vi "MouseScrollAction.vi"(0 "XYGraph输入":refnum<vi>, 1 "Ynum":i32=8, 2 "Coords":T2, 3 "Delta":i32, 4 "PlatMods":T1, 5 "ZoomMode":u16) -> ()   [LabVIEW 2015]
uses:
  <vilib>/Utility/miscctls.llb/LVPoint32TypeDef.ctl
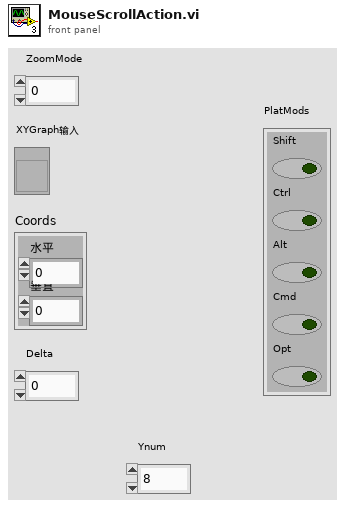
[diagram p1: front panel]
types:
  T1 = cluster{"Shift":bool, "Ctrl":bool, "Alt":bool, "Cmd":bool, "Opt":bool}
  T2 = typedef "LVPoint32TypeDef.ctl" = cluster{"Horizontal":i32, "Vertical":i32}
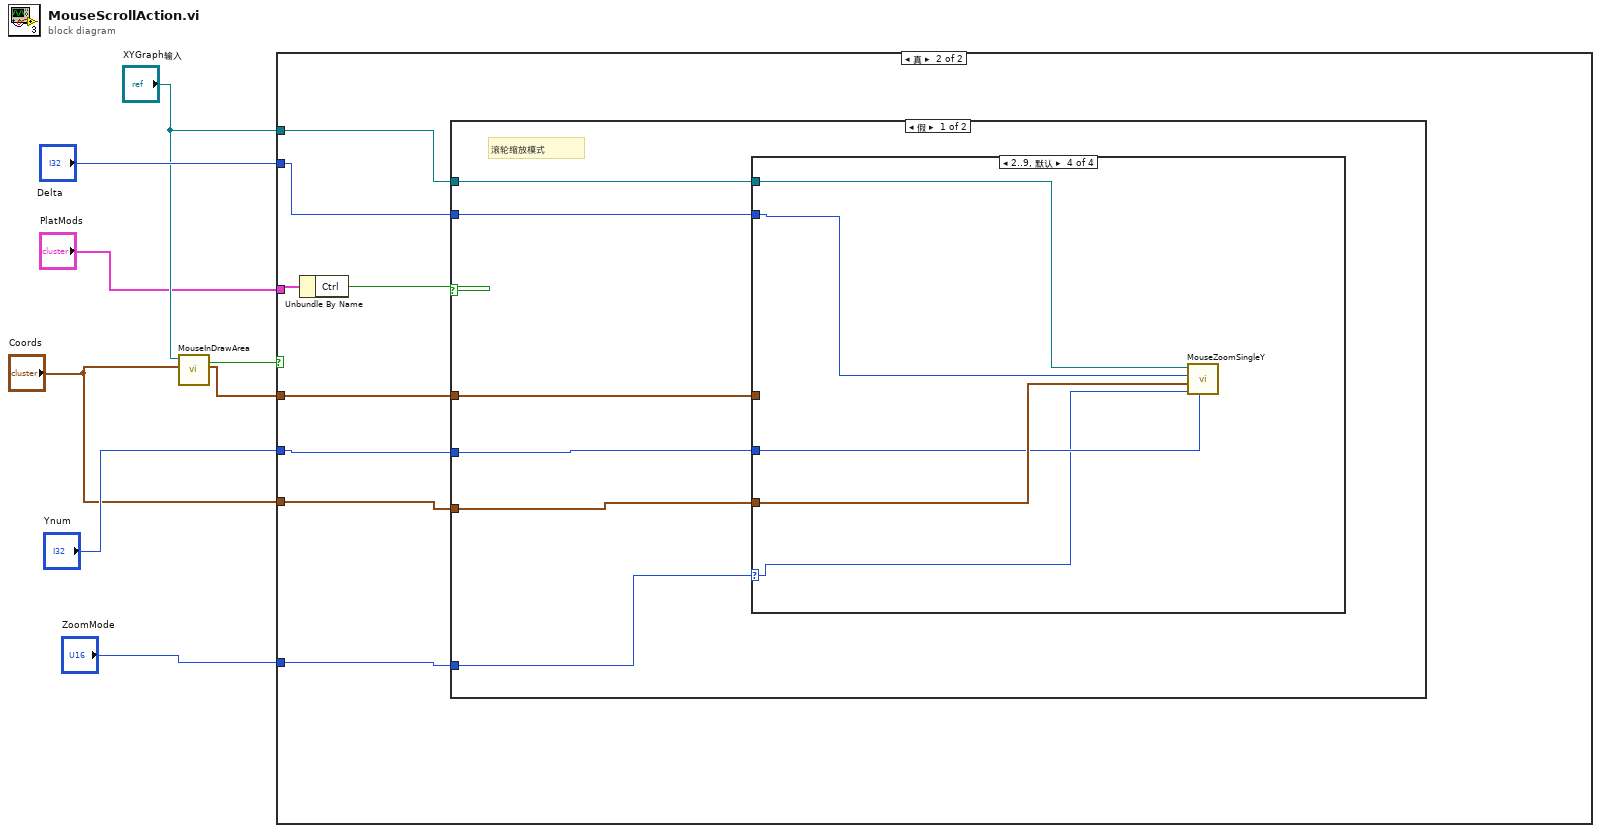
[diagram p0: block diagram]
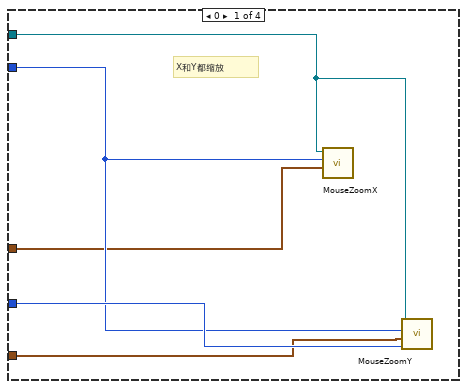
[diagram p3: hidden frame]
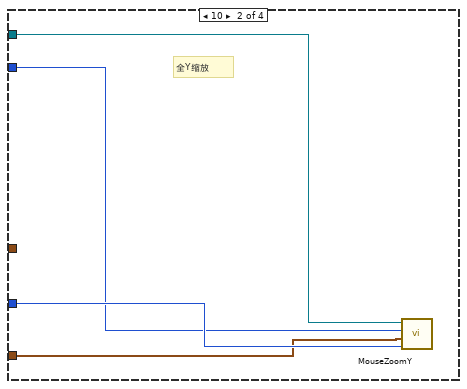
[diagram p4: hidden frame]
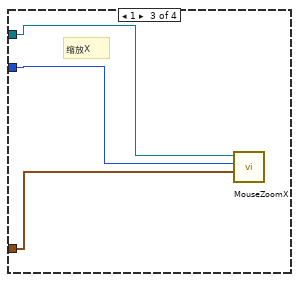
[diagram p5: hidden frame]
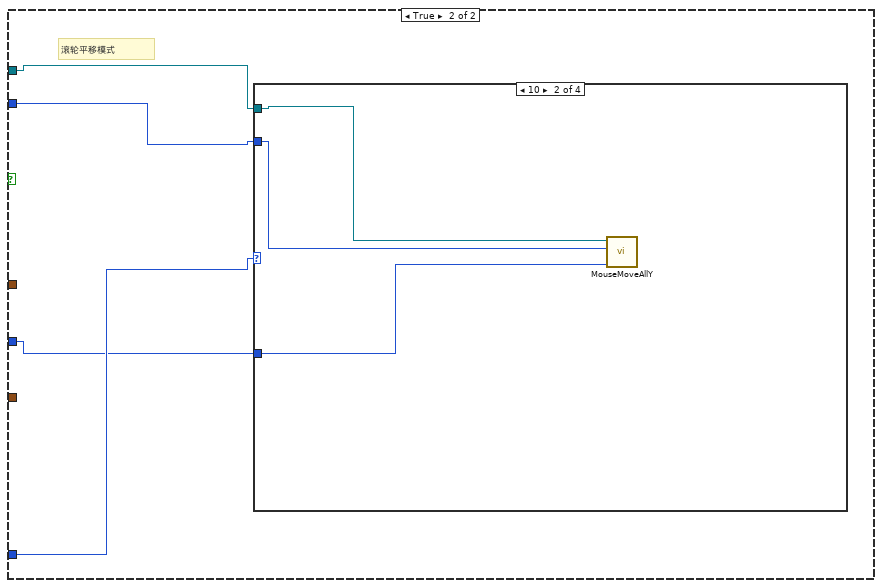
[diagram p6: hidden frame]
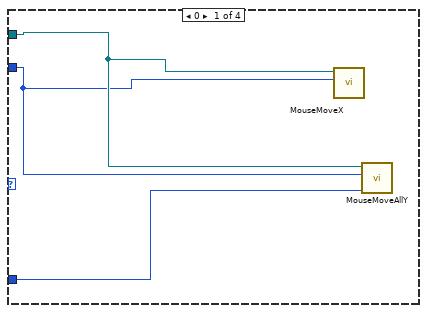
[diagram p7: hidden frame]
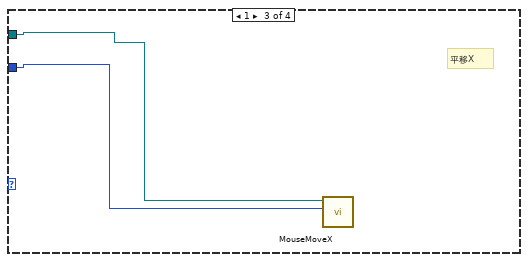
[diagram p8: hidden frame]
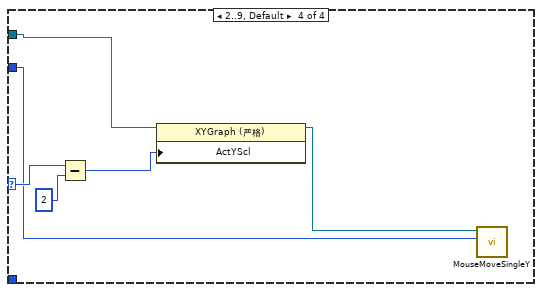
[diagram p9: hidden frame]
diagram:
  n1 = call "MouseInDrawArea.vi"("Coords"="Coords", "XYGraph输入"="XYGraph输入") -> ("InOrNot"=w4:bool, "XY"=w5:cluster{"X":dbl, "Y":dbl})  [unwired: 7 in]
  n2 = case shown="真" w4 {
    tunnel: "PlatMods" -> [_ w16]
    tunnel: "XYGraph输入" -> [_ w15]
    tunnel: "Delta" -> [_ w14]
    tunnel: w5 -> [_ w13]
    tunnel: "Coords" -> [_ w12]
    tunnel: "ZoomMode" -> [_ w11]
    tunnel: "Ynum" -> [_ w10]
    frame False {
    }
    frame True {
      n3 = Unbundle By Name(w16) -> ("Ctrl"=w9:bool)
      n4 = case shown="假" w9 {
        tunnel: w15 -> [w21 w42]
        tunnel: w14 -> [w20 w41]
        tunnel: w13 -> [w19 _]
        tunnel: w12 -> [w18 _]
        tunnel: w10 -> [w22 w40]
        tunnel: w11 -> [w17 w43]
        frame False {
          # "滚轮缩放模式"
          n5 = case shown="2..9, 默认" w17 {
            selector: w17 -> [_ _ _ w35]
            tunnel: w22 -> [w27 w31 _ w38]
            tunnel: w21 -> [w26 w30 w34 w36]
            tunnel: w20 -> [w25 w29 w33 w37]
            tunnel: w19 -> [w24 _ w32 _]
            tunnel: w18 -> [w23 w28 _ w39]
            frame 0 {
              # "X和Y都缩放"
              n6 = call "MouseZoomX.vi"("XY"=w24, "Delta"=w25, "XYGraph输入"=w26) -> ()  [unwired: 9 in]
              n7 = call "MouseZoomY.vi"("YNum"=w27, "Coords"=w23, "Delta"=w25, "XYGraph输入"=w26) -> ()  [unwired: 8 in]
            }
            frame 10 {
              # "全Y缩放"
              n8 = call "MouseZoomY.vi"("YNum"=w31, "Coords"=w28, "Delta"=w29, "XYGraph输入"=w30) -> ()  [unwired: 8 in]
            }
            frame 1 {
              # "缩放X"
              n9 = call "MouseZoomX.vi"("XY"=w32, "Delta"=w33, "XYGraph输入"=w34) -> ()  [unwired: 9 in]
            }
            frame 2..9, Default {
              n10 = call "MouseZoomSingleY.vi"("YNum"=w38, "ZoomMode"=w35, "Coords"=w39, "Delta"=w37, "XYGraph输入"=w36) -> ()  [unwired: 7 in]
            }
          }
        }
        frame True {
          # "滚轮平移模式"
          n11 = case shown="10" w43 {
            selector: w43 -> [_ _ _ w56]
            tunnel: w42 -> [w45 w49 w51 w57]
            tunnel: w41 -> [w44 w47 w50 w52]
            tunnel: w40 -> [w46 w48 _ _]
            frame 0 {
              n12 = call "MouseMoveX.vi"("Delta"=w44, "XYGraph输入"=w45) -> ()  [unwired: 10 in]
              n13 = call "MouseMoveAllY.vi"("YNum"=w46, "Delta"=w44, "XYGraph输入"=w45) -> ()  [unwired: 9 in]
            }
            frame 10 {
              n14 = call "MouseMoveAllY.vi"("YNum"=w48, "Delta"=w47, "XYGraph输入"=w49) -> ()  [unwired: 9 in]
            }
            frame 1 {
              # "平移X"
              n15 = call "MouseMoveX.vi"("Delta"=w50, "XYGraph输入"=w51) -> ()  [unwired: 10 in]
            }
            frame 2..9, Default {
              n16 = Subtract(x=w56, y=u16 2) -> (x-y=w54:u16)
              n17 = property class="XYGraph (严格)"(reference=w57, "ActYScl"=w54) -> (reference out=w53:refnum<vi>)  [unwired: 1 in, 1 out]
              n18 = call "MouseMoveSingleY.vi"("Delta"=w52, "XYGraph输入"=w53) -> ()  [unwired: 10 in]
            }
          }
        }
      }
    }
  }
